vi "Modbus PLC Comm Tester.vi"() -> ()   [LabVIEW 2018]
uses:
  MB PLC Client.lvclass
  Data/MB Data Block.lvclass
  Types/TCP Config_Cluster.ctl
  MB PLC Client.lvlib
  Types/MB Ref Range_Cluster.ctl
  Types/PLC Config_Cluster.ctl
  Types/Serial Config_Cluster.ctl
  <vilib>/Plasmionique/MB Master/MB_Master/MB_Master.lvclass
  <vilib>/Plasmionique/MB Master/MB_ADU/MB_ADU.lvclass
panel:
  out "Last Error Time":string
  in  "Tab Control 2":T1(tab)
  in  "Swap Words":bool
  in  "Reference Format":u16(ring)=5 items=["4 Digits"=4, "5 Digits"=5, "6 Digits"=6]
  in  "Open":bool
  in  "Close":bool
  in  "Type":enum16{"Serial", "TCP"}(ring) caption="Connection Type"
  in  "Tab Control":enum32{"Page 1", "Page 2"}(tab)
  in  "Retries":u8=1
  in  "Timeout (ms)":u32=300
  in  "Flow Control":u16(ring) items=["None", "XON/XOFF", "RTS/CTS", "XON/XOFF & RTS/CTS", "DTR/DSR", "XON/XOFF & DTR/DSR"]
  in  "Parity":u16(ring) items=["None", "Odd", "Even", "Mark", "Space"]
  in  "Stop Bits":u16(ring)=10 items=["1.0"=10, "1.5"=15, "2.0"=20]
  in  "Baud Rate (bps)":u32(ring)=19200 items=["9600"=9600, "19200"=19200, "38400"=38400, "57600"=57600, "115200"=115200, "460800"=460800, "921600"=921600]
  in  "Slave Address":u8=1
  in  "Mode":enum16{"RTU", "ASCII"}(ring)
  in  "COM Port":refnum<visa-resource-name>
  in  "TCP_Port":u16=502 caption="Port"
  in  "IP Address":string="localhost"
  in  "TCP_Timeout":i32=10000 caption="Timeout (ms)"
  in  "TCP_Slave ID":u8=255 caption="Slave ID" format="%.0x"
  in  "Poll Period (ms)":i32=100
  out "Message Log":T2(array[cluster]) {"dt" format="%d ms"; "Time" format="%<%.0X %x>T"}
  out "Last Error Status":errorcluster
  in  "Edit 2":bool
  in  "Remove":bool
  in  "Edit":bool
  in  "Add":bool
  in  "Watchlist":i32(listbox)
  out "Input Registers":u16[](array[numeric])
  out "Holding Registers":u16[](array[numeric])
  out "Discrete Inputs":bool[](array[boolean])
  out "Coils":bool[](array[boolean])
  out "Open?":bool caption="Connected"
  # "Communication Settngs"
  # "Communication Status"
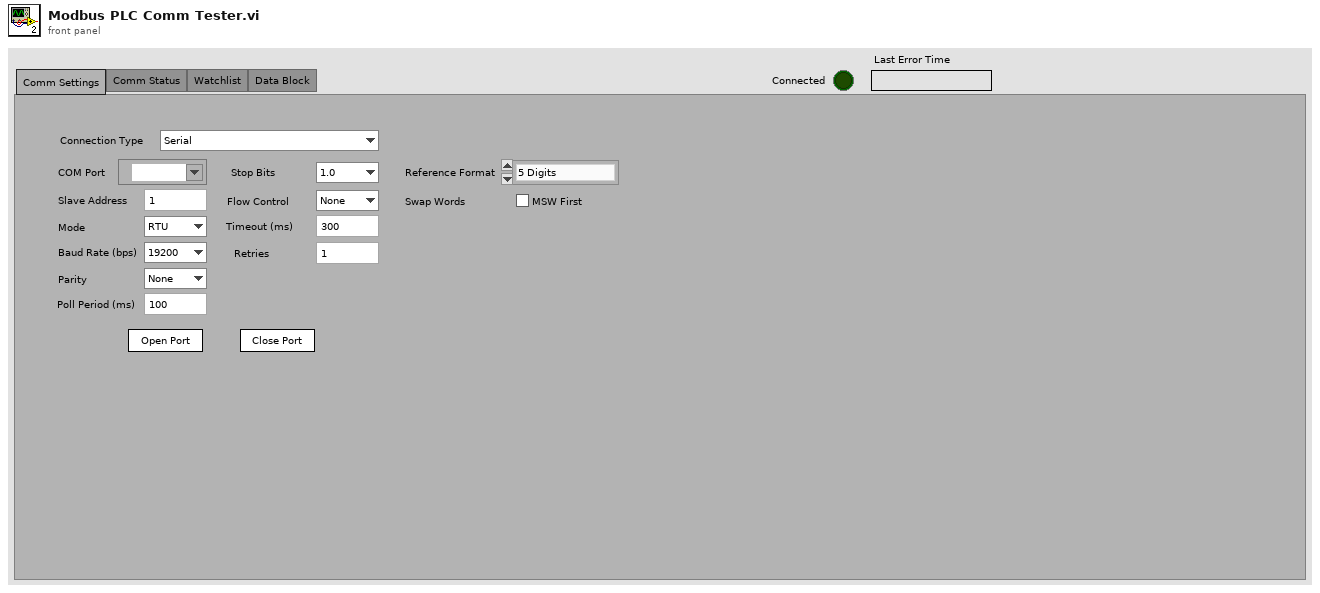
[diagram p1: front panel]
types:
  T1 = enum32{"Comm Settings", "Comm Status", "Watchlist", "Data Block"}
  T2 = cluster{"Time":timestamp, "TX":string, "RX":string, "dt":dbl}[]
  T3 = cluster{"Timestamp":timestamp, "TX":string, "RX":string, "dt":u32}
  T4 = typedef "MB PLC Client.lvlib/Serial Config_Cluster.ctl" = cluster{"COM Port":string, "Slave ID":u8, "baud rate (bps)":u32, "Mode":enum16{"RTU", "ASCII"}, "Parity":u16, "Flow Control":u16, "Timeout":u32, "Retries":u8, "Stop Bits":u16}
  T5 = typedef "MB PLC Client.lvlib/PLC Config_Cluster.ctl" = cluster{"Use TCP":bool, "Reference Format":u16, "Swap Words":bool, "Poll List":T6[]}
  T6 = typedef "MB PLC Client.lvlib/MB Ref Range_Cluster.ctl" = cluster{"Start":u32, "Qty":u16}
  T7 = typedef "MB PLC Client.lvlib/TCP Config_Cluster.ctl" = cluster{"IP Address":string, "Port":u16, "Slave ID":i8, "Timeout":i32}
  T8 = cluster{"Properties:TX Timestamp":timestamp, "string":string, "string":string, u32}
  T9 = cluster{"Timestamp":timestamp, "TX":string, "RX":string, "dt":u32}[]
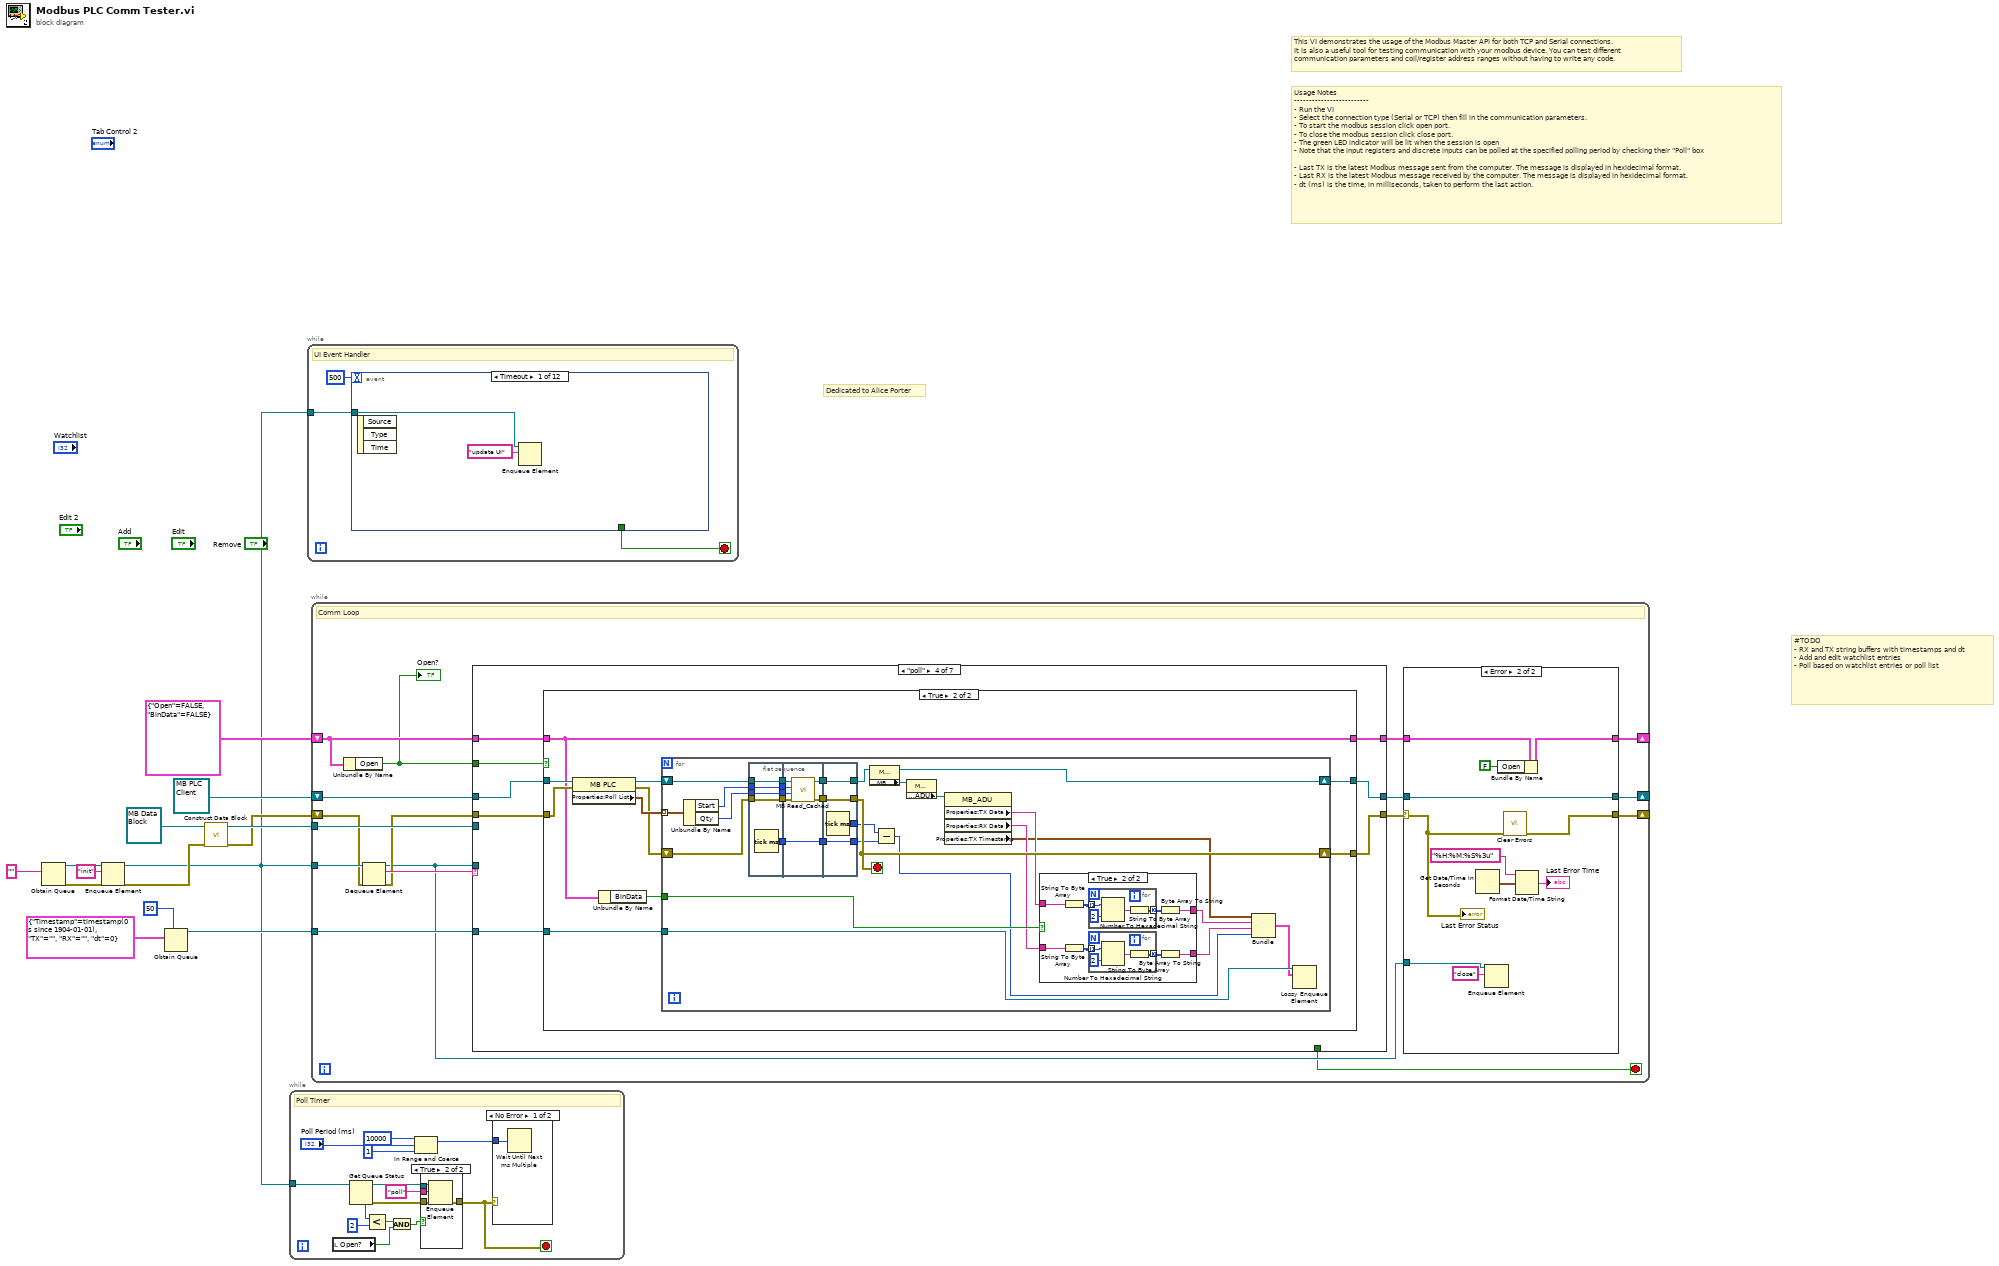
[diagram p0: block diagram]
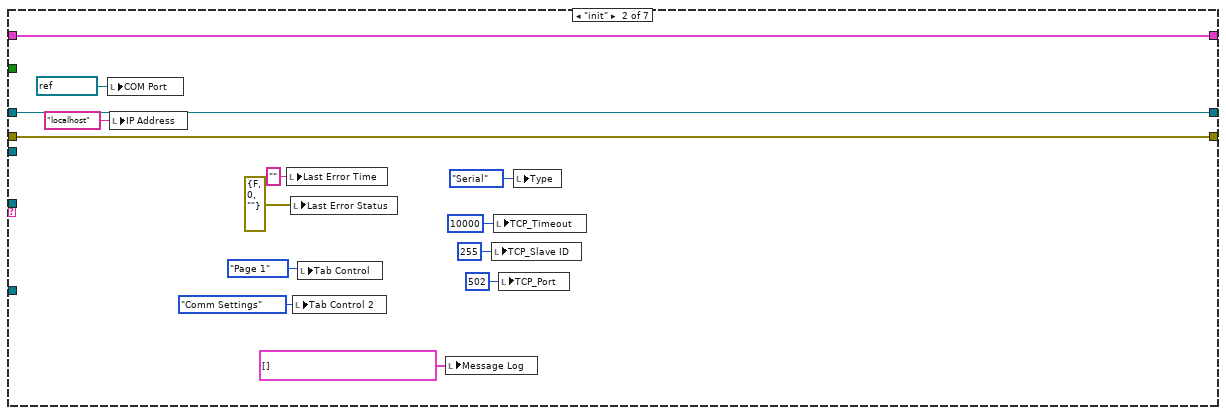
[diagram p6: hidden frame]
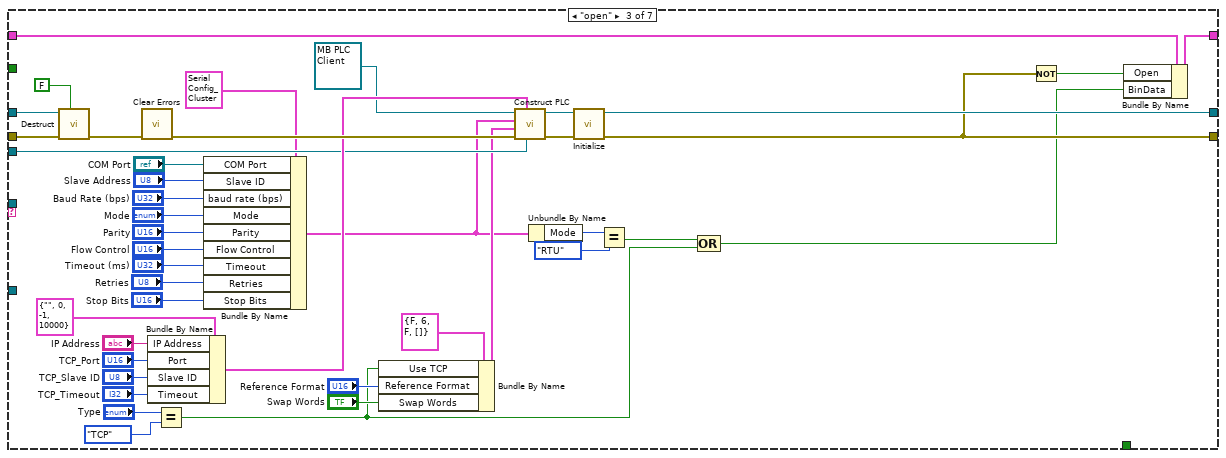
[diagram p7: hidden frame]
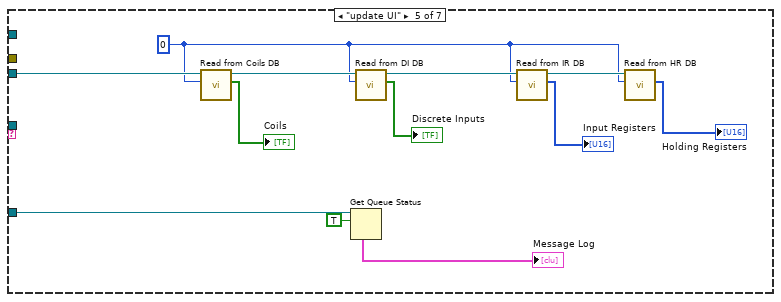
[diagram p10: hidden frame]
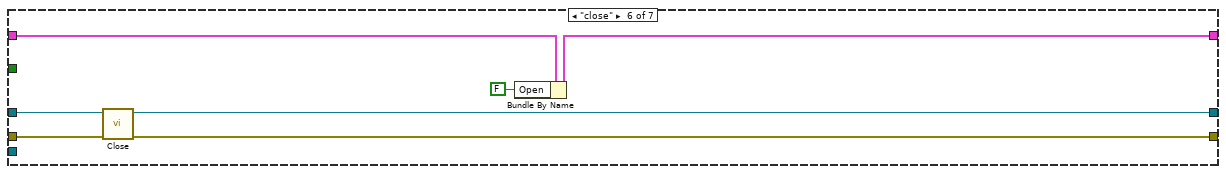
[diagram p11: hidden frame]
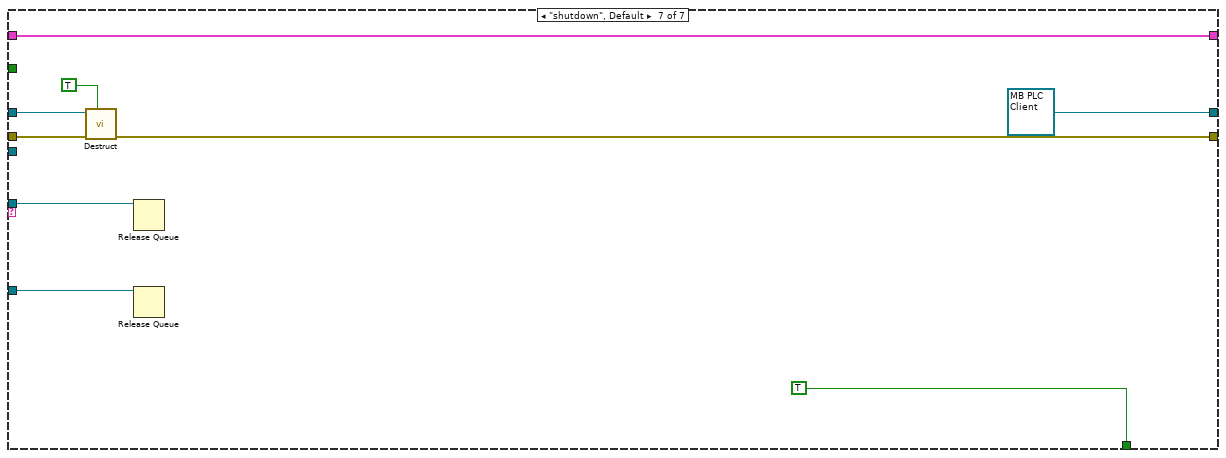
[diagram p12: hidden frame]
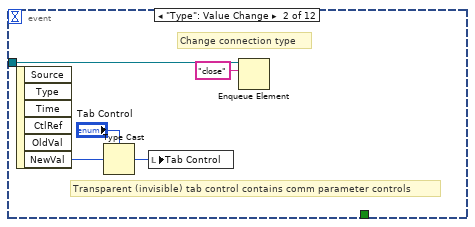
[diagram p13: hidden frame]
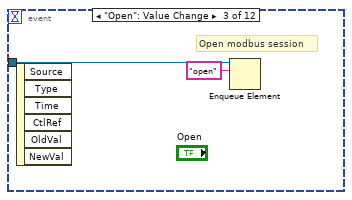
[diagram p14: hidden frame]
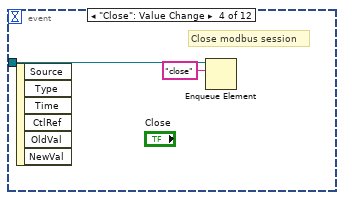
[diagram p15: hidden frame]
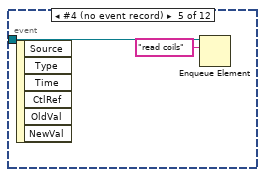
[diagram p16: hidden frame]
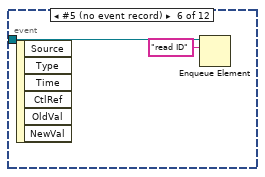
[diagram p17: hidden frame]
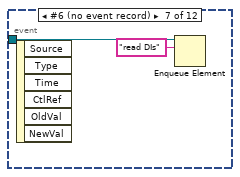
[diagram p18: hidden frame]
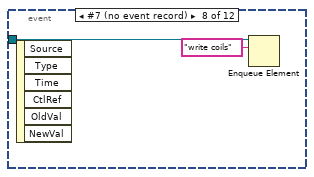
[diagram p19: hidden frame]
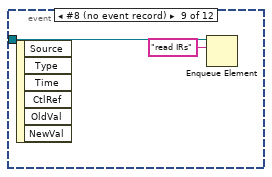
[diagram p20: hidden frame]
diagram:
  # "Dedicated to Alice Porter"
  # "#TODO\n- RX and TX string buffers with timestamps and dt\n- Add and edit watchlist entries\n- Poll based on watchlist entries or poll list"
  # "Usage Notes\n-------------------------\n- Run the VI\n- Select the connection type (Serial or TCP) then fill in the communication parameters.\n- To start the modbus session click open port.\n- To close the modbus session click close port.\n- The green LED indicator will be lit when the session is open\n- Note that the input registers and discrete inputs can be polled at the specified polling period by checking their \"Poll\" box\n\n- Last TX is the latest Modbus message sent from the computer. The message is displayed in hexidecimal format.\n- Last RX is the latest Modbus message received by the computer. The message is displayed in hexidecimal format. \n- dt (ms) is the time, in milliseconds, taken to perform the last action."
  # "This VI demonstrates the usage of the Modbus Master API for both TCP and Serial connections.\nIt is also a useful tool for testing communication with your modbus device. You can test different\ncommunication parameters and coil/register address ranges without having to write any code."
  n1 = Obtain Queue(element data type="") -> (queue out=w8:refnum<queue>, error out=w10:errorcluster)  [unwired: 4 in, 1 out]
  n2 = Enqueue Element(queue=w8, element="init", error in (no error)=w10) -> (queue out=w1:refnum<queue>, error out=w6:errorcluster)  [unwired: 1 in, 1 out]
  n3 = Obtain Queue(max queue size (-1, unlimited)=50, element data type=T3 {"Timestamp"=timestamp(0 s since 1904-01-01), "TX"="", "RX"="", "dt"=0}) -> (queue out=w2:refnum<queue>)  [unwired: 3 in, 2 out]
  n4 = call-dynamic "Construct Data Block.vi"("error in (no error)"=w6, "Modbus Data Store in"=refnum<class "MB Data Block.lvclass"> refnum ("MB Data Block (default)")) -> ("error out"=w5:errorcluster, "Modbus Data Store out"=w12:refnum<class "MB Data Block.lvclass">)  [unwired: 8 in]
  n5 = while {
    tunnel: w1 -> [w28]
    stop <- w19 stop-if-true
    # "Poll Timer"
    n6 = local read "Open?"() -> (w16:bool)
    n7 = Get Queue Status(queue=w28) -> (queue out=w20:refnum<queue>, error out=w21:errorcluster, # elements in queue=w27:i32)  [unwired: 2 in, 5 out]
    n8 = Less?(x=w27, y=2) -> (x < y?=w17:bool)
    n9 = And(x=w17, y=w16) -> (x .and. y?=w15:bool)
    n10 = In Range and Coerce(upper limit=10000, x="Poll Period (ms)", lower limit=1) -> (coerced(x)=w22:i32)  [unwired: 1 out]
    n11 = case shown="True" w15 {
      tunnel: w21 -> [w29 w33]
      tunnel: w20 -> [_ w32]
      tunnel: [w29 w31] -> w19
      tunnel: "poll" -> [_ w30]
      frame False {
      }
      frame True {
        n12 = Enqueue Element(queue=w32, element=w30, error in (no error)=w33) -> (error out=w31:errorcluster)  [unwired: 1 in, 2 out]
      }
    }
    n13 = case shown="No Error" w19 {
      tunnel: w22 -> [w34 _]
      frame No Error {
        n14 = Wait Until Next ms Multiple(millisecond multiple=w34) -> ()  [unwired: 1 out]
      }
      frame Error {
      }
    }
  }
  n15 = while {
    tunnel: w1 -> [w37]
    stop <- w36 stop-if-true
    # "UI Event Handler"
    n16 = event shown="[0] Timeout" {
      selector: _ -> [_ _ _ _ _ _ _ _ _ _ _ _]
      dyn-events: _ -> [_ _ _ _ _ _ _ _ _ _ _ _]
      timeout: 500 -> [_ _ _ _ _ _ _ _ _ _ _ _]
      tunnel: w37 -> [w38 w43 w46 w47 w49 w51 w53 w55 w57 w59 w61 w63]
      tunnel: [_ _ _ _ _ _ _ _ _ _ _ TRUE] -> w36
      event Timeout {
        n17 = event-data() -> ()  [unwired: 1 in, 3 out]
        n18 = Enqueue Element(queue=w38, element="update UI") -> ()  [unwired: 2 in, 3 out]
      }
      event "Type": Value Change {
        # "Transparent (invisible) tab control contains comm parameter controls"
        # "Change connection type"
        n19 = event-data() -> ("NewVal"=w42:enum16{"Serial", "TCP"})  [unwired: 1 in, 5 out]
        n20 = Type Cast(type="Tab Control", x=w42) -> (*(type *) &x=w40:enum32{"Page 1", "Page 2"})
        n21 = local write "Tab Control"(w40) -> ()
        n22 = Enqueue Element(queue=w43, element="close") -> ()  [unwired: 2 in, 3 out]
      }
      event "Open": Value Change {
        # "Open modbus session"
        n23 = event-data() -> ()  [unwired: 1 in, 6 out]
        n24 = Enqueue Element(queue=w46, element="open") -> ()  [unwired: 2 in, 3 out]
      }
      event "Close": Value Change {
        # "Close modbus session"
        n25 = event-data() -> ()  [unwired: 1 in, 6 out]
        n26 = Enqueue Element(queue=w47, element="close") -> ()  [unwired: 2 in, 3 out]
      }
      event #4 (no event record) {
        n27 = event-data() -> ()  [unwired: 1 in, 6 out]
        n28 = Enqueue Element(queue=w49, element="read coils") -> ()  [unwired: 2 in, 3 out]
      }
      event #5 (no event record) {
        n29 = event-data() -> ()  [unwired: 1 in, 6 out]
        n30 = Enqueue Element(queue=w51, element="read ID") -> ()  [unwired: 2 in, 3 out]
      }
      event #6 (no event record) {
        n31 = event-data() -> ()  [unwired: 1 in, 6 out]
        n32 = Enqueue Element(queue=w53, element="read DIs") -> ()  [unwired: 2 in, 3 out]
      }
      event #7 (no event record) {
        n33 = event-data() -> ()  [unwired: 1 in, 6 out]
        n34 = Enqueue Element(queue=w55, element="write coils") -> ()  [unwired: 2 in, 3 out]
      }
      event #8 (no event record) {
        n35 = event-data() -> ()  [unwired: 1 in, 6 out]
        n36 = Enqueue Element(queue=w57, element="read IRs") -> ()  [unwired: 2 in, 3 out]
      }
      event #9 (no event record) {
        n37 = event-data() -> ()  [unwired: 1 in, 6 out]
        n38 = Enqueue Element(queue=w59, element="read HRs") -> ()  [unwired: 2 in, 3 out]
      }
      event #10 (no event record) {
        n39 = event-data() -> ()  [unwired: 1 in, 6 out]
        n40 = Enqueue Element(queue=w61, element="write HRs") -> ()  [unwired: 2 in, 3 out]
      }
      event Panel Close? {
        n41 = event-data() -> ()  [unwired: 1 in, 4 out]
        n42 = Enqueue Element(queue=w63, element="shutdown") -> ()  [unwired: 2 in, 3 out]
        n43 = event-data("Discard?"=TRUE) -> ()  [unwired: 1 in, 1 out]
      }
    }
  }
  n44 = while {
    shift-right: [w68] -> _
    shift-left: refnum<class "MB PLC Client.lvclass"> refnum ("PLC in") -> [w83]
    tunnel: w12 -> [w82]
    shift-right: [w71] -> _
    shift-left: w5 -> [w73]
    shift-right: [w69] -> _
    shift-left: cluster{"Open":bool, "BinData":bool} {"Open"=FALSE, "BinData"=FALSE} -> [w80]
    tunnel: w1 -> [w81]
    tunnel: w2 -> [w78]
    stop <- w67 stop-if-true
    # "Comm Loop"
    n45 = Unbundle By Name(w80) -> ("Open"=w79:bool)
    "Open?" <- w79
    n46 = Dequeue Element(queue=w81, error in (no error)=w73) -> (queue out=w70:refnum<queue>, element=w77:string, error out=w72:errorcluster)  [unwired: 1 in, 1 out]
    n47 = case shown="\"poll\"" w77 {
      tunnel: w83 -> [w98 w103 w146 w163 _ w255 w265]
      tunnel: w82 -> [_ _ w143 _ w248 _ _]
      tunnel: [w98 w103 w136 w161 _ w254 refnum<class "MB PLC Client.lvclass"> refnum ("PLC out")] -> w74
      tunnel: [w99 w102 w122 w160 _ w253 w261] -> w76
      tunnel: w80 -> [w100 w104 w124 w159 _ w258 w266]
      tunnel: [w100 w104 w123 w158 _ w256 w266] -> w75
      tunnel: w72 -> [w99 w102 w121 w162 _ w252 w264]
      tunnel: w70 -> [_ _ _ _ _ _ w260]
      tunnel: w79 -> [_ _ _ w164 _ _ _]
      tunnel: w78 -> [_ _ _ w157 w251 _ w259]
      tunnel: [_ _ _ _ _ _ TRUE] -> w67
      frame "set poll list" {
      }
      frame "init" {
        n48 = local write "COM Port"(refnum<visa-resource-name> refnum ("COM Port")) -> ()
        n49 = local write "IP Address"("localhost" ("IP Address")) -> ()
        n50 = local write "Last Error Time"("" ("Last Error Time")) -> ()
        n51 = local write "Last Error Status"(errorcluster {"status"=FALSE, "code"=0, "source"=""} ("Last Error Status")) -> ()
        n52 = local write "Tab Control 2"(enum32{"Comm Settings", "Comm Status"}."Comm Settings" ("Tab Control 2")) -> ()
        n53 = local write "Tab Control"(enum32{"Page 1", "Page 2"}."Page 1" ("Tab Control")) -> ()
        n54 = local write "Message Log"(T2 [] ("Message Log")) -> ()
        n55 = local write "TCP_Slave ID"(u8 255 ("TCP_Slave ID")) -> ()
        n56 = local write "TCP_Timeout"(10000 ("TCP_Timeout")) -> ()
        n57 = local write "TCP_Port"(u16 502 ("TCP_Port")) -> ()
        n58 = local write "Type"(enum16{"Serial", "TCP"}."Serial" ("Type")) -> ()
      }
      frame "open" {
        n59 = call-dynamic "Destruct.vi"("Destroy Data Block? (t)"=FALSE, "error in (no error)"=w121, "PLC in"=w146) -> ("error out"=w145:errorcluster)  [unwired: 8 in]
        n60 = call <vilib>:"Clear Errors.vi"("error in (no error)"=w145) -> ("error out"=w154:errorcluster)  [unwired: 5 in, 1 out]
        n61 = Bundle By Name(cluster=T7 {"IP Address"="", "Port"=0, "Slave ID"=-1, "Timeout"=10000} ("TCP Config"), "IP Address"="IP Address", "Port"="TCP_Port", "Slave ID"="TCP_Slave ID", "Timeout"="TCP_Timeout") -> (w148:T7)
        n62 = Equal?(x="Type", y=enum16{"Serial", "TCP"}."TCP") -> (x = y?=w116:bool)
        n63 = Bundle By Name(cluster=T4 {"COM Port"="COM1", "Slave ID"=1, "baud rate (bps)"=460800, "Mode"=enum."RTU", "Parity"=0, "Flow Control"=0, "Timeout"=200, "Retries"=1, "Stop Bits"=10} ("Serial Config"), "COM Port"="COM Port", "Slave ID"="Slave Address", "baud rate (bps)"="Baud Rate (bps)", "Mode"="Mode", "Parity"="Parity", "Flow Control"="Flow Control", "Timeout"="Timeout (ms)", "Retries"="Retries", "Stop Bits"="Stop Bits") -> (w120:T4)
        n64 = Bundle By Name(cluster=T5 {"Use TCP"=FALSE, "Reference Format"=6, "Swap Words"=FALSE, "Poll List"=[]} ("PLC Config"), "Use TCP"=w116, "Reference Format"="Reference Format", "Swap Words"="Swap Words") -> (w139:T5)
        n65 = call-dynamic "Construct PLC.vi"("MB Data Block (default)"=w143, "TCP Config"=w148, "error in (no error)"=w154, "PLC Config"=w139, "Serial Config"=w120, "PLC in"=refnum<class "MB PLC Client.lvclass"> refnum) -> ("error out"=w140:errorcluster, "PLC out"=w141:refnum<class "MB PLC Client.lvclass">)  [unwired: 4 in]
        n66 = Unbundle By Name(w120) -> ("Mode"=w119:enum16{"RTU", "ASCII"})
        n67 = call-dynamic "Initialize.vi"("error in (no error)"=w140, "PLC in"=w141) -> ("error out"=w122:errorcluster, "PLC out"=w136:refnum<class "MB PLC Client.lvclass">)  [unwired: 8 in]
        n68 = Equal?(x=w119, y=enum16{"RTU", "ASCII"}."RTU") -> (x = y?=w117:bool)
        n69 = Compound Arithmetic op=OR(w117, w116) -> (w115:bool)
        n70 = Not(x=w122) -> (.not. x?=w125:bool)
        n71 = Bundle By Name(cluster=w124, "Open"=w125, "BinData"=w115) -> (w123:cluster{"Open":bool, "BinData":bool})
      }
      frame "poll" {
        n72 = case shown="True" w164 {
          tunnel: w163 -> [w166 w174]
          tunnel: [w166 w176] -> w161
          tunnel: [w165 w175] -> w160
          tunnel: w162 -> [w165 w171]
          tunnel: w159 -> [_ w169]
          tunnel: [_ w169] -> w158
          tunnel: w157 -> [_ w167]
          frame False {
          }
          frame True {
            n73 = property class="MB PLC"(reference=w174, error in=w171) -> (reference out=w173:refnum<class "MB PLC Client.lvclass">, error out=w170:errorcluster, "Properties:Poll List"=w172:T6[])
            n74 = Unbundle By Name(w169) -> ("BinData"=w168:bool)
            n75 = for {
              shift-right: [w186] -> w176
              shift-left: w173 -> [w205]
              tunnel: w172 -> [w204] mode=indexing
              shift-right: [w200] -> w175
              shift-left: w170 -> [w201]
              tunnel: w168 -> [w184]
              tunnel: w167 -> [w178]
              stop <- w200 stop-if-true
              n76 = Unbundle By Name(w204) -> ("Start"=w203:u32, "Qty"=w202:u16)
              n77 = flat-sequence {
                tunnel: w201 -> [w225]
                tunnel: w202 -> [w226]
                tunnel: w203 -> [w227]
                tunnel: w205 -> [w228]
                tunnel: [w228] -> w199
                tunnel: [w227] -> w198
                tunnel: [w226] -> w197
                tunnel: [w225] -> w196
                tunnel: [w224] -> w192
                tunnel: w199 -> [w235]
                tunnel: w198 -> [w233]
                tunnel: w197 -> [w232]
                tunnel: w196 -> [w231]
                tunnel: [w234] -> w195
                tunnel: [w230] -> w194
                tunnel: [w229] -> w193
                tunnel: w192 -> [w229]
                tunnel: [w238] -> w200
                tunnel: [w239] -> w191
                tunnel: w195 -> [w239]
                tunnel: w194 -> [w238]
                tunnel: [w237] -> w187
                tunnel: w193 -> [w237]
                tunnel: [w236] -> w188
                frame #0 {
                  n78 = Tick Count (ms)() -> (millisecond timer value=w224:u32)
                }
                frame #1 {
                  n79 = call "MB Read_Cached.vi"("error in (no error)"=w231, "Quantity(1)"=w232, "Modbus Reference"=w233, "MB PLC in"=w235) -> ("error out"=w230:errorcluster, "MB PLC out"=w234:refnum<class "MB PLC Client.lvclass">)  [unwired: 6 in]
                }
                frame #2 {
                  n80 = Tick Count (ms)() -> (millisecond timer value=w236:u32)
                }
              }
              n81 = property class="MB PLC"(reference=w191) -> (reference out=w186:refnum<class "MB PLC Client.lvclass">, "Properties:MB session"=w190:refnum<class "MB_Master.lvclass">)  [unwired: 1 in, 1 out]
              n82 = Subtract(x=w188, y=w187) -> (x-y=w179:u32)
              n83 = property class="MB_Master"(reference=w190) -> ("Properties:ADU"=w189:refnum<class "MB_ADU.lvclass">)  [unwired: 1 in, 2 out]
              n84 = property class="MB_ADU"(reference=w189) -> ("Properties:TX Data"=w185:string, "Properties:RX Data"=w183:string, "Properties:TX Timestamp"=w181:timestamp)  [unwired: 1 in, 2 out]
              n85 = case shown="True" w184 {
                tunnel: w185 -> [w207 w211]
                tunnel: w183 -> [w206 w210]
                tunnel: [w207 w209] -> w182
                tunnel: [w206 w208] -> w180
                frame False {
                }
                frame True {
                  n86 = String To Byte Array(string=w211) -> (unsigned byte array=w214:u8[])
                  n87 = String To Byte Array(string=w210) -> (unsigned byte array=w213:u8[])
                  n88 = for {
                    tunnel: w214 -> [w223] mode=indexing
                    tunnel: [w221] -> w215 mode=concatenating
                    n89 = Number To Hexadecimal String(1:i16 2 ("width (-)"), 2:w223) -> (0:w220:string)
                    n90 = String To Byte Array(string=w220) -> (unsigned byte array=w221:u8[])
                  }
                  n91 = for {
                    tunnel: w213 -> [w219] mode=indexing
                    tunnel: [w217] -> w212 mode=concatenating
                    n92 = Number To Hexadecimal String(1:i16 2 ("width (-)"), 2:w219) -> (0:w216:string)
                    n93 = String To Byte Array(string=w216) -> (unsigned byte array=w217:u8[])
                  }
                  n94 = Byte Array To String(unsigned byte array=w215) -> (string=w209:string)
                  n95 = Byte Array To String(unsigned byte array=w212) -> (string=w208:string)
                }
              }
              n96 = Bundle("Properties:TX Timestamp"=w181, "string"=w182, "string"=w180, w179) -> (w177:T8)  [unwired: 1 in]
              n97 = Lossy Enqueue Element(queue=w178, element=w177) -> ()  [unwired: 1 in, 4 out]
            }
          }
        }
      }
      frame "update UI" {
        w240 = u16 0 ("Modbus Address")
        n98 = call-dynamic "Read from Coils DB.vi"("Modbus Address"=w240, "MB Data Block in"=w248) -> ("Data out"=→"Coils":bool[], "MB Data Block out"=w247:refnum<class "MB Data Block.lvclass">)  [unwired: 7 in, 1 out]
        n99 = Get Queue Status(queue=w251, return elements? (F)=TRUE) -> (elements=→"Message Log":T9)  [unwired: 1 in, 7 out]
        n100 = call-dynamic "Read from DI DB.vi"("Modbus Address"=w240, "MB Data Block in"=w247) -> ("Data out"=→"Discrete Inputs":bool[], "MB Data Block out"=w244:refnum<class "MB Data Block.lvclass">)  [unwired: 7 in, 1 out]
        n101 = call-dynamic "Read from IR DB.vi"("Modbus Address"=w240, "MB Data Block in"=w244) -> ("Data out"=→"Input Registers":u16[], "MB Data Block out"=w243:refnum<class "MB Data Block.lvclass">)  [unwired: 7 in, 1 out]
        n102 = call-dynamic "Read from HR DB.vi"("Modbus Address"=w240, "MB Data Block in"=w243) -> ("Data out"=→"Holding Registers":u16[])  [unwired: 7 in, 2 out]
      }
      frame "close" {
        n103 = call-dynamic "Close.vi"("error in (no error)"=w252, "PLC in"=w255) -> ("error out"=w253:errorcluster, "PLC out"=w254:refnum<class "MB PLC Client.lvclass">)  [unwired: 8 in]
        n104 = Bundle By Name(cluster=w258, "Open"=FALSE) -> (w256:cluster{"Open":bool, "BinData":bool})
      }
      frame "shutdown", Default {
        n105 = call-dynamic "Destruct.vi"("Destroy Data Block? (t)"=TRUE, "error in (no error)"=w264, "PLC in"=w265) -> ("error out"=w261:errorcluster)  [unwired: 8 in]
        n106 = Release Queue(queue=w260) -> ()  [unwired: 2 in, 3 out]
        n107 = Release Queue(queue=w259) -> ()  [unwired: 2 in, 3 out]
      }
    }
    n108 = case shown="Error" w76 {
      selector: w76 -> [w84 w93]
      tunnel: w75 -> [w86 w90]
      tunnel: w74 -> [w85 w87]
      tunnel: [w84 w92] -> w71
      tunnel: w70 -> [_ w91]
      tunnel: [w86 w88] -> w69
      tunnel: [w85 w87] -> w68
      frame No Error {
      }
      frame Error {
        n109 = Get Date/Time In Seconds() -> (seconds since 1Jan1904=w97:timestamp)
        n110 = Enqueue Element(queue=w91, element="close") -> ()  [unwired: 2 in, 3 out]
        n111 = Bundle By Name(cluster=w90, "Open"=FALSE) -> (w88:cluster{"Open":bool, "BinData":bool})
        n112 = call <vilib>:"Clear Errors.vi"("error in (no error)"=w93) -> ("error out"=w92:errorcluster)  [unwired: 5 in, 1 out]
        n113 = Format Date/Time String(time format string (%c)="%H:%M:%S%3u", seconds (now)=w97) -> (date/time string=→"Last Error Time":string)  [unwired: 1 in]
        "Last Error Status" <- w93
      }
    }
  }
